vi "CALCULO_CHECKSUM_SUB.vi"(1 "DATOS":string) -> (0 "verificado":string)   [LabVIEW 2017]
panel:
  out "XOR":u32
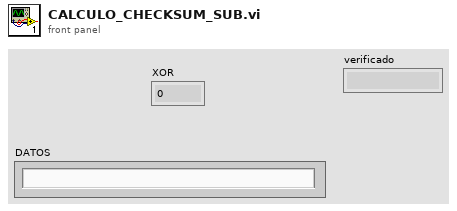
[diagram p1: front panel]
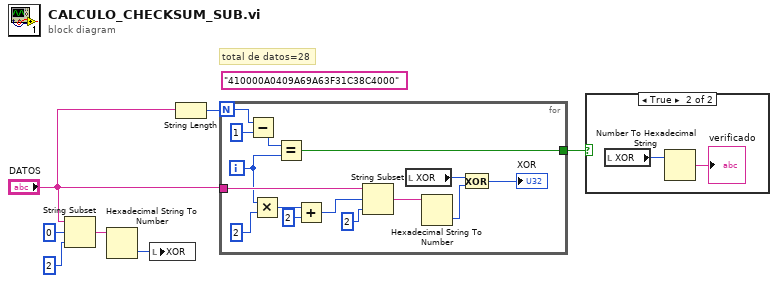
[diagram p0: block diagram]
diagram:
  (unwired) "410000A0409A69A63F31C38C4000" ("DATOS")
  # "total de datos=28"
  n1 = String Subset(string="DATOS", offset (0)=0, length (rest)=2 ("length (rest)")) -> (substring=w7:string)
  n2 = Hexadecimal String To Number(string=w7) -> (number=w5:u32)  [unwired: 2 in, 1 out]
  n3 = local write "XOR"(w5) -> ()
  n4 = String Length(string="DATOS") -> (length=w2:i32)
  n5 = for {
    N: w2 -> [w13]
    tunnel: "DATOS" -> [w14]
    tunnel: [w8] -> w1
    i -> [w9]
    n6 = Subtract(x=w13, y=1) -> (x-y=w10:i32)
    n7 = Multiply(x=w9, y=2) -> (x*y=w17:i32)
    n8 = Equal?(x=w10, y=w9) -> (x = y?=w8:bool)
    n9 = Add(x=w17, y=2) -> (x+y=w16:i32)
    n10 = String Subset(string=w14, offset (0)=w16, length (rest)=2 ("length (rest)")) -> (substring=w21:string)
    n11 = local read "XOR"() -> (w20:u32)
    n12 = Hexadecimal String To Number(string=w21) -> (number=w19:u32)  [unwired: 2 in, 1 out]
    n13 = Exclusive Or(1:w19, 2:w20) -> (0:→"XOR":u32)
  }
  n14 = case shown="True" w1 {
    frame False {
    }
    frame True {
      n15 = local read "XOR"() -> (w24:u32)
      n16 = Number To Hexadecimal String(2:w24) -> (0:→"verificado":string)  [unwired: 1 in]
    }
  }
